vi "Focus Move Relative.vi"(8 "error in (no error)":errorcluster, 9 "Counts":i32, 10 "Motor (0:n-1)":i32, 11 "Focus Class in":refnum<class "Focus Class.lvclass">) -> (0 "error out":errorcluster, 2 "response":string, 3 "Focus Class out":refnum<class "Focus Class.lvclass">)   [LabVIEW 2024, in "Focus Class.lvclass"]
uses:
  Focus Class.lvclass
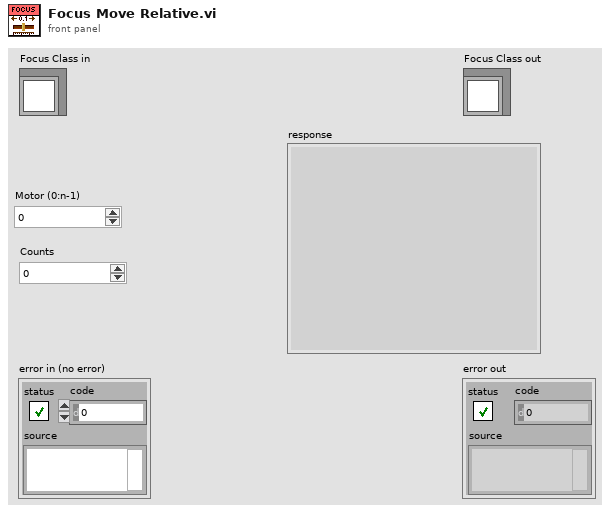
[diagram p1: front panel]
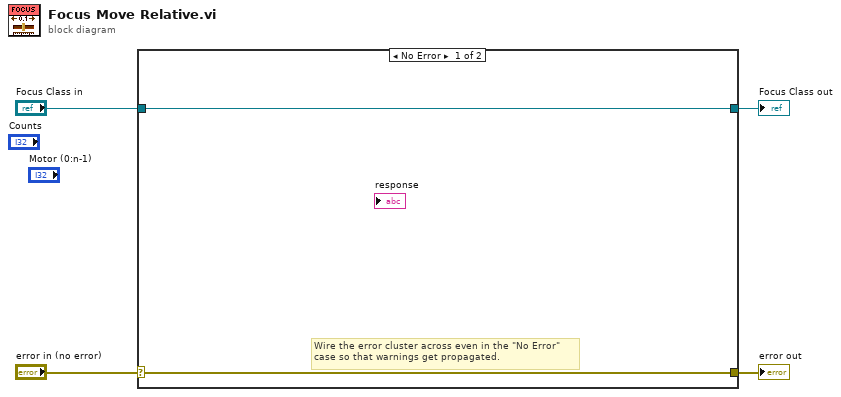
[diagram p0: block diagram]
diagram:
  n1 = case shown="No Error" "error in (no error)" {
    selector: "error in (no error)" -> [w5 w8]
    tunnel: [w5 w8] -> w3
    tunnel: [w6 w7] -> w1
    tunnel: "Focus Class in" -> [w6 w7]
    frame No Error {
      # "Wire the error cluster across even in the \"No Error\"\ncase so that warnings get propagated."
    }
    frame Error {
    }
  }
  "error out" <- w3
  "Focus Class out" <- w1
